vi "Fenster anpassen.vi"(9 "Trennbalken":refnum<vi>[](array[refnum]), 10 "Tabelle":refnum<vi>, 11 "vi reference":refnum<vi>) -> (3 "Fehler (Ausgang)":errorcluster)   [LabVIEW 2020, in "FT-IR.lvlib" / "Spanfaktor.lvlib"]
uses:
  Spanfaktor.lvlib
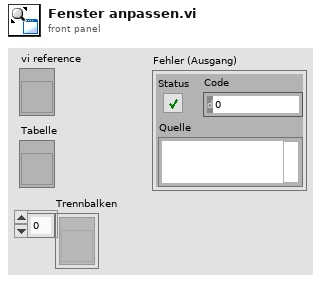
[diagram p1: front panel]
types:
  T1 = typedef "LVRectTypeDef.ctl" = cluster{"Left":i16, "Top":i16, "Right":i16, "Bottom":i16}
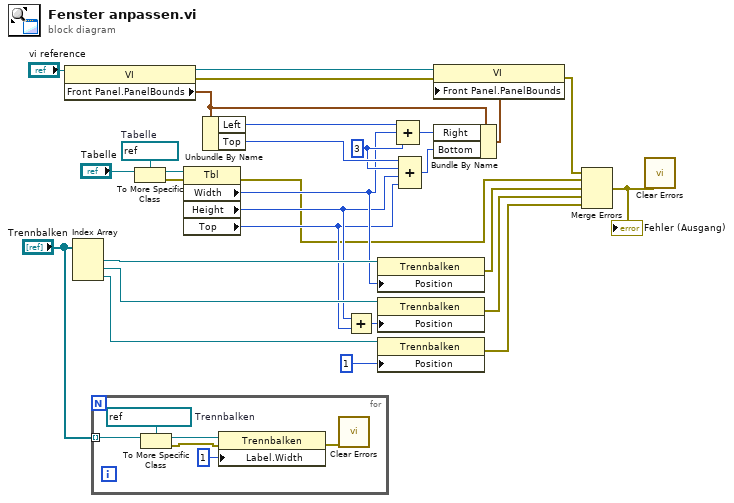
[diagram p0: block diagram]
diagram:
  w18 = u32 3 ("Wert")
  w29 = refnum<vi> refnum  # Tabelle
  n1 = property class="VI"(reference="vi reference") -> (reference out=w19:refnum<vi>, error out=w26:errorcluster, "Front Panel.PanelBounds"=w22:T1)  [unwired: 1 in]
  n2 = Index Array(array="Trennbalken") -> (element #1=w17:refnum<vi>, element #2=w16:refnum<vi>, element #3=w15:refnum<vi>)  [unwired: 3 in]
  n3 = for {
    tunnel: "Trennbalken" -> [w30] mode=indexing
    w33 = refnum<vi> refnum  # Trennbalken
    n4 = To More Specific Class(target class=w33, reference=w30) -> (specific class reference=w31:refnum<vi>, error out=w32:errorcluster)  [unwired: 1 in]
    n5 = property class="Trennbalken"(reference=w31, error in=w32, "Label.Width"=u32 1 ("Beschriftung.Größe:Breite")) -> (error out=w34:errorcluster)  [unwired: 1 out]
    n6 = call <vilib>:"Clear Errors.vi"("error in (no error)"=w34) -> ()  [unwired: 5 in, 2 out]
  }
  n7 = To More Specific Class(target class=w29, reference="Tabelle") -> (specific class reference=w28:refnum<vi>, error out=w27:errorcluster)  [unwired: 1 in]
  n8 = property class="Tbl"(reference=w28, error in=w27) -> (error out=w1:errorcluster, "Width"=w14:u32, "Height"=w12:u32, "Top"=w11:i32)  [unwired: 1 out]
  n9 = Unbundle By Name(w22) -> ("Left"=w20:i16, "Top"=w21:i16)
  n10 = Add(x=w12, y=w11) -> (x+y=w13:u32)
  n11 = property on="Eigenschaftsknoten" class="Trennbalken"(reference=w17, "Position"=w14) -> (error out=w8:errorcluster)  [unwired: 1 in, 1 out]
  n12 = property on="Eigenschaftsknoten" class="Trennbalken"(reference=w16, "Position"=w13) -> (error out=w7:errorcluster)  [unwired: 1 in, 1 out]
  n13 = property on="Eigenschaftsknoten" class="Trennbalken"(reference=w15, "Position"=1 ("Trennbalkenposition")) -> (error out=w6:errorcluster)  [unwired: 1 in, 1 out]
  n14 = Compound Arithmetic op=ADD(w20, w14, w18) -> (w23:u32)
  n15 = Compound Arithmetic op=ADD(w21, w18, w12, w11) -> (w24:u32)
  n16 = Bundle By Name(cluster=w22, "Right"=w23, "Bottom"=w24) -> (w25:T1)
  n17 = property class="VI"(reference=w19, error in=w26, "Front Panel.PanelBounds"=w25) -> (error out=w9:errorcluster)  [unwired: 1 out]
  n18 = Merge Errors(w9, w1, w8, w7, w6) -> (w5:errorcluster)
  "Fehler (Ausgang)" <- w5
  n19 = call <vilib>:"Clear Errors.vi"("error in (no error)"=w5) -> ()  [unwired: 5 in, 2 out]
